vi "Current times Temp Fault.vi"(5 "Resistance":T1 format="%_6g", 6 "Max Temp":T1 format="%_6g", 7 "Coil Voltage":T1 format="%_6g", 9 "Temp Coef":T1 format="%_6g", 10 "Current":T1 format="%_6g", 11 "Inductive V":T1 format="%_6g") -> (3 "I * Temp Fault":bool)   [LabVIEW 2017]
doc: "Author: Scott Hannahs <sth@magnet.fsu.edu>\nCopyright 2018 Florida State University, All rights reserved."
uses:
  SCH Data Controls/SCH Data 2 RT.ctl
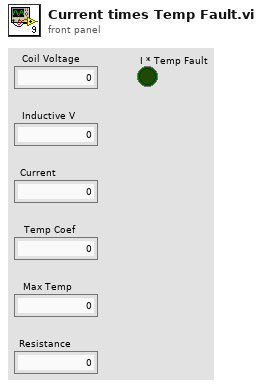
[diagram p1: front panel]
types:
  T1 = typedef "SCH Data 2 RT.ctl" = fxp<+/-,38,12>
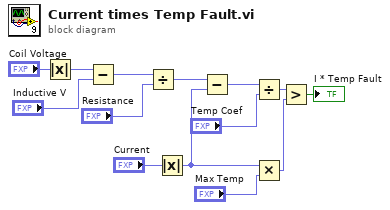
[diagram p0: block diagram]
diagram:
  n1 = Absolute Value(x="Coil Voltage") -> (abs(x)=w2:fxp<+,38,12>)
  n2 = Subtract(x=w2, y="Inductive V") -> (x-y=w5:T1)
  n3 = Divide(x=w5, y="Resistance") -> (x/y=w7:T1)
  n4 = Absolute Value(x="Current") -> (abs(x)=w1:fxp<+,38,12>)
  n5 = Subtract(x=w7, y=w1) -> (x-y=w8:T1)
  n6 = Divide(x=w8, y="Temp Coef") -> (x/y=w9:fxp<+/-,34,10>)
  n7 = Multiply(x=w1, y="Max Temp") -> (x*y=w14:T1)
  n8 = Greater?(x=w9, y=w14) -> (0:→"I * Temp Fault":bool)
